vi "Generate Sine SweepV3.vi"() -> ()   [LabVIEW 2018]
uses:
  <vilib>/addons/_NISVFA/_Shared subVIs/Controls/svc_Channel Info.ctl
  <vilib>/addons/_NISVFA/_Shared subVIs/Controls/svc_Engineering Units Text Ring.ctl
  <vilib>/addons/_NISVFA/_Shared subVIs/Controls/svc_Weighting Filter Text Ring.ctl
  <vilib>/sound2/lvsound2.llb/Sound Output Task ID.ctl
  <vilib>/sound2/lvsound2.llb/Sound Input Task ID.ctl
  <vilib>/sound2/lvsound2.llb/Sound Data Format.ctl
  <vilib>/sound2/lvsound2.llb/Sampling Mode.ctl
  <vilib>/addons/Sound and Vibration/svt_Calibration/SVL Scale Voltage to EU (1 Ch).vi
  <vilib>/addons/_NISVFA/_Shared subVIs/Common/svc_Set SV Channel Info.vi
  <vilib>/addons/_NISVFA/_Shared subVIs/Common/svc_Set SV Channel Info (variant).vi
  <vilib>/addons/_NISVFA/_Shared subVIs/Common/SVL Set dB Reference (variant).vi
  <vilib>/sound2/lvsound2.llb/Sound Output Set Volume (Single).vi
  <vilib>/sound2/lvsound2.llb/Sound Output Write (DBL Single).vi
  <vilib>/sound2/lvsound2.llb/Sound Input Read (DBL).vi
  <vilib>/sound2/lvsound2.llb/Sound File Write Open.vi
  <vilib>/sound2/lvsound2.llb/Sound File Write (DBL Single).vi
  <vilib>/addons/_NISVFA/_Shared subVIs/Common/svc_Engineering Units to Unit Label.vi
  <vilib>/addons/_NISVFA/_Shared subVIs/Common/svc_Compute Scale Factor to Convert V to EU.vi
  <vilib>/addons/_NISVFA/_Shared subVIs/Common/svc_Compute Scale Factor to Convert C to EU.vi
  <vilib>/addons/_NISVFA/_Shared subVIs/Common/svc_Set dB ref if Pascal.vi
  <vilib>/addons/_NISVFA/_Shared subVIs/Common/svc_Caller VI Returned in Error Source.vi
  <vilib>/measure/maspectr.llb/FFT Power Spectrum and PSD for 1 Chan.vi
  <vilib>/addons/_NISVFA/_Baseband FFT/SVFA Frequency Response (1x1) (Mag-Phase).vi
  <vilib>/measure/macond.llb/FIR Filter for 1 Chan.vi
  <vilib>/Analysis/3filter.llb/Butterworth Filter (DBL).vi
  <vilib>/addons/_NISVFA/_Generation/SoundVib_Generation.lvlib
  <vilib>/addons/Sound and Vibration/svt_Calibration/SoundVib_Calibration.lvlib
  <vilib>/Analysis/NI_AALBase.lvlib
  <vilib>/measure/NI_MAPro.lvlib
  Program Files (x86)/National Instruments/LabVIEW 2018/examples/Sound and Vibration/SoundVib_Audio Examples.lvlib
panel:
  in  "Data Dir":path
  out "aligned signals length":i32
  out "FFT 2":cluster{"f0":dbl, "df":dbl, "magnitude":dbl[]}(graph)
  out "FFT":cluster{"f0":dbl, "df":dbl, "magnitude":dbl[]}(graph)
  in  "averaging parameters 2":T1={"averaging mode"=enum."RMS averaging", "weighting mode"=enum."Exponential", "number of averages"=10, "linear mode"=enum."Auto restart"}
  in  "FRF mode":enum16{"H1", "H2", "H3"}(ring)
  in  "view":T2={"dB On (T)"=TRUE, "unwrap phase (F)"=FALSE, "convert to degree (T)"=TRUE}
  in  "channel info Mic":T3={"sensor sensitivity"=1000.0, "engineering units"=1, "dB reference"=1.0, "custom label"="EU", "weighting filter"=0, "pregain"=0.0} {"pregain" format="%.2f"; "weighting filter" items=["Linear", "A-weighting", "B-weighting", "C-weighting", "ITU-R 468-4", "Dolby", "CCITT", "C-message", "Wb", "Wc", "Wd", "We", "Wf", "Wh", "Wj", "Wk", "Wm", "AES17 20 kHz lowpass", "AES17 40 kHz lowpass", "AES17 20 kHz highpass", "AES17 40 kHz highpass"]; "dB reference" format="%^.1e"; "engineering units" items=["custom..."=0, "V"=1, "A"=21, "C"=30, "pC"=31, "s"=32, "-"=29, "Pa"=2, "N"=20, "g"=3, "m/s^2"=4, "m/s"=5, "m"=6, "mm/s"=12, "mm"=13, "micron/s"=14, "micron"=15, "in/s^2"=7, "in/s"=8, "in"=9, "mil/s"=10, "mil"=11, "rad/s^2"=16, "rad/s"=17, "rad"=18, "deg/s^2"=26, "deg/s"=27, "deg"=28, "RPM"=22, "cycle/s^2"=23, "Hz"=24, "cycle"=25, "strain"=19]; "sensor sensitivity" format="%#_5f"}
  in  "channel info Spk":T3={"sensor sensitivity"=1000.0, "engineering units"=1, "dB reference"=1.0, "custom label"="EU", "weighting filter"=0, "pregain"=0.0} {"pregain" format="%.2f"; "weighting filter" items=["Linear", "A-weighting", "B-weighting", "C-weighting", "ITU-R 468-4", "Dolby", "CCITT", "C-message", "Wb", "Wc", "Wd", "We", "Wf", "Wh", "Wj", "Wk", "Wm", "AES17 20 kHz lowpass", "AES17 40 kHz lowpass", "AES17 20 kHz highpass", "AES17 40 kHz highpass"]; "dB reference" format="%^.1e"; "engineering units" items=["custom..."=0, "V"=1, "A"=21, "C"=30, "pC"=31, "s"=32, "-"=29, "Pa"=2, "N"=20, "g"=3, "m/s^2"=4, "m/s"=5, "m"=6, "mm/s"=12, "mm"=13, "micron/s"=14, "micron"=15, "in/s^2"=7, "in/s"=8, "in"=9, "mil/s"=10, "mil"=11, "rad/s^2"=16, "rad/s"=17, "rad"=18, "deg/s^2"=26, "deg/s"=27, "deg"=28, "RPM"=22, "cycle/s^2"=23, "Hz"=24, "cycle"=25, "strain"=19]; "sensor sensitivity" format="%#_5f"}
  out "error out 2":errorcluster
  out "FRF":cluster{"f0":dbl, "df":dbl, "magnitude":dbl[]}(graph)
  out "Waveform Mic":waveform(dbl)[](graph)
  in  "error in (no error)":errorcluster
  in  "Samples/Sec":dbl=44100.0
  in  "Amplitude":dbl(slide)=1.0 min=0.0 max=1.0 scale=0.0..1.0
  in  "device In":u32
  out "Dur(s)":dbl
  out "error out":errorcluster
  in  "device Out":u32
  in  "Duration[s]":dbl=3.0
  in  "Freq Spacing":enum16{"Linear", "Logarithmic"}(ring)=enum."Logarithmic"
  out "Waveform Out":waveform(dbl)(graph)
  in  "frequency range [Hz]":cluster{"start":dbl, "stop":dbl}={"start"=20.0, "stop"=20000.0} {"stop" format="%.2f"; "start" format="%.2f"}
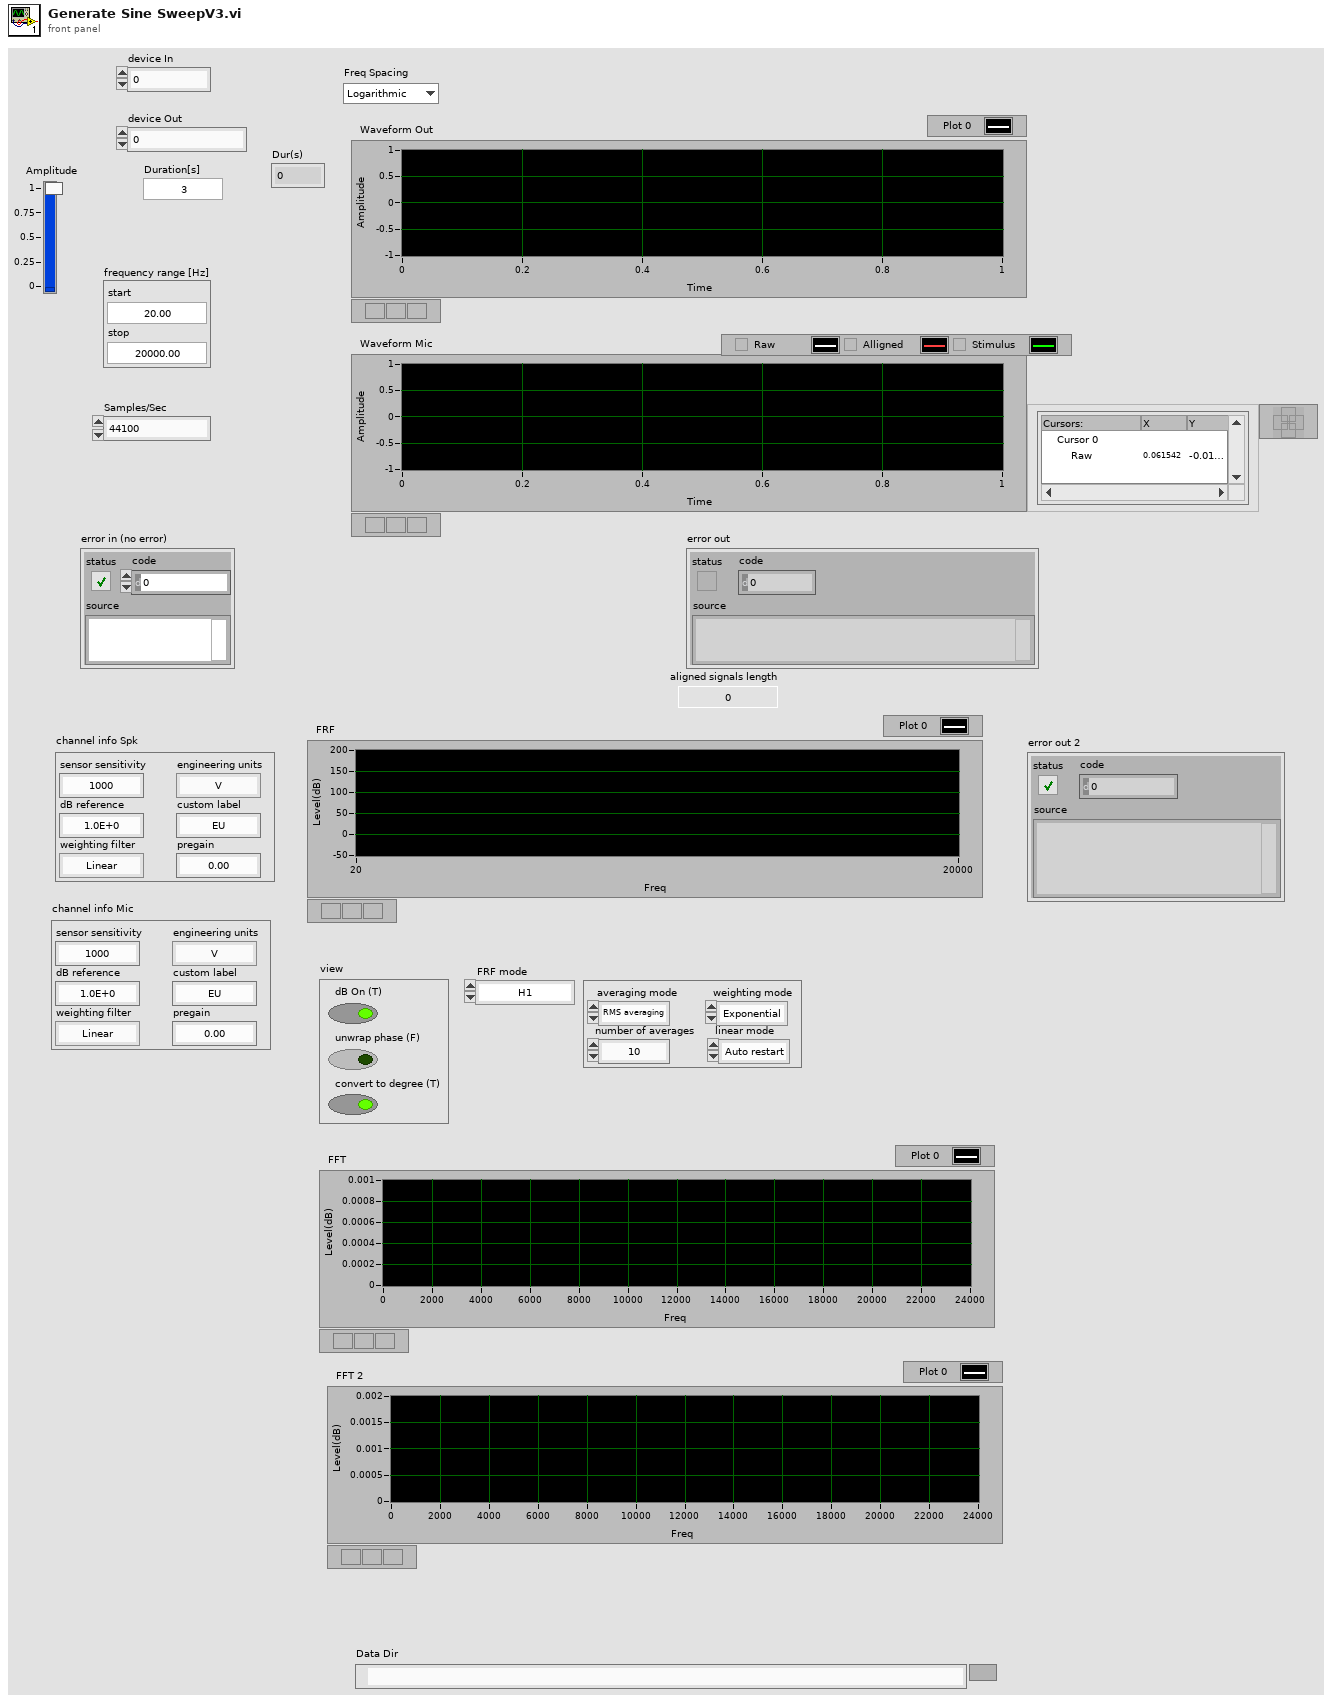
[diagram p1: front panel]
types:
  T1 = cluster{"averaging mode":enum16{"No averaging", "Vector averaging", "RMS averaging", "Peak hold"}, "weighting mode":enum16{"Linear", "Exponential"}, "number of averages":u32, "linear mode":enum16{"One shot", "Auto restart"}}
  T2 = cluster{"dB On (T)":bool, "unwrap phase (F)":bool, "convert to degree (T)":bool}
  T3 = typedef "svc_Channel Info.ctl" = cluster{"sensor sensitivity":dbl, "engineering units":T4, "dB reference":dbl, "custom label":string, "weighting filter":T5, "pregain":dbl}
  T4 = typedef "svc_Engineering Units Text Ring.ctl" = u16
  T5 = typedef "svc_Weighting Filter Text Ring.ctl" = u16
  T6 = typedef "Sound Data Format.ctl" = cluster{"sample rate (S/s)":dbl, "number of channels":i32, "bits per sample":i32}
  T7 = cluster{"Topology":enum16{"Off", "FIR by Specification", "Equi-ripple FIR", "Windowed FIR"}, "Type":enum16{"Lowpass", "Highpass", "Bandpass", "Bandstop"}, "#Taps":i32, "Lower PB":dbl, "Upper PB":dbl, "Lower SB":dbl, "Upper SB":dbl}
  T8 = typedef "Sound Input Task ID.ctl" = u32
  T9 = typedef "Sound Output Task ID.ctl" = u32
  T10 = cluster{"Start":dbl, "TaskPlay":T9, "TaskMic":T8, "SampleInfo":cluster{"Fs":dbl, "#s":u32}, "Waveform":waveform(dbl), "Samples/Sec":dbl, "Duration[s]":dbl, "Mic":waveform(dbl)[], "RcdSmpl":i32, "SoundFmt":T6}
  T11 = typedef "Sampling Mode.ctl" = i32
  T12 = typedef "Sound File Refnum.ctl" = refnum<file>
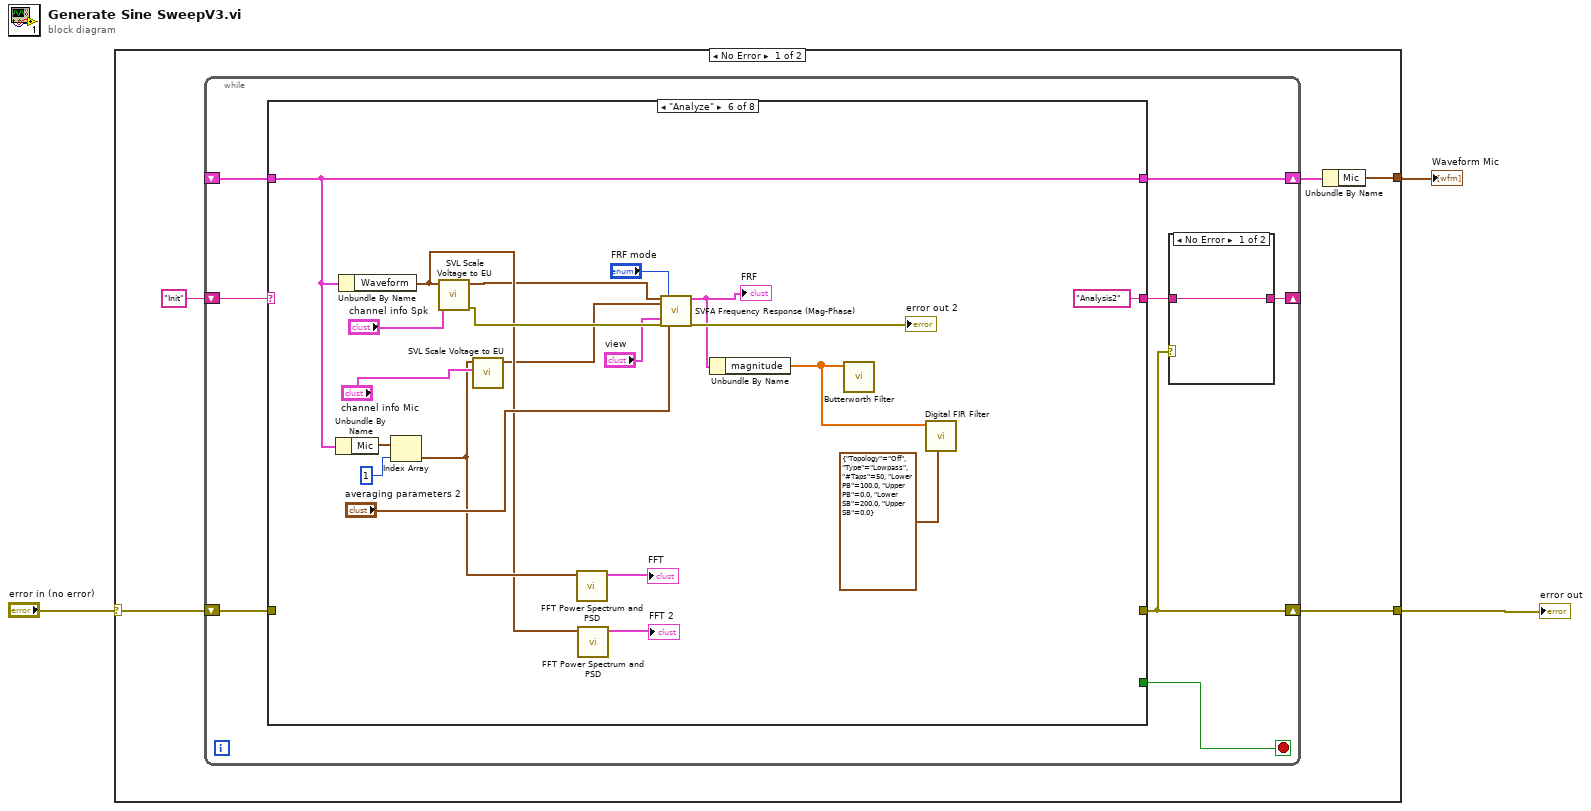
[diagram p0: block diagram]
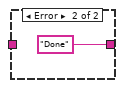
[diagram p2: hidden frame]
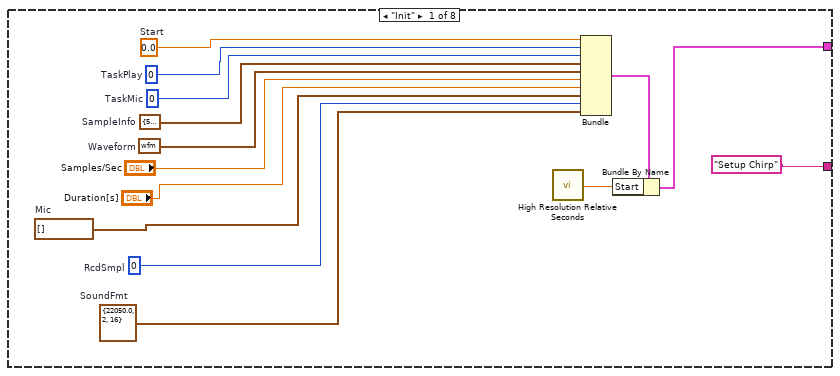
[diagram p3: hidden frame]
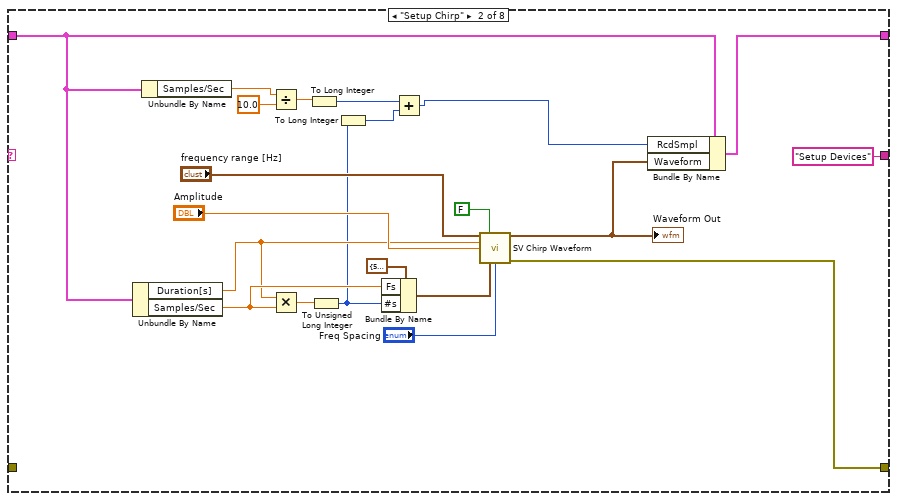
[diagram p4: hidden frame]
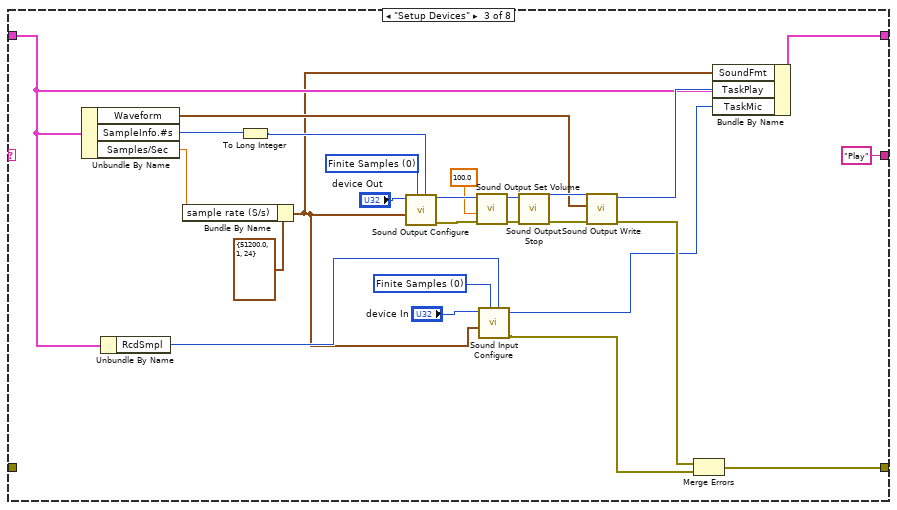
[diagram p5: hidden frame]
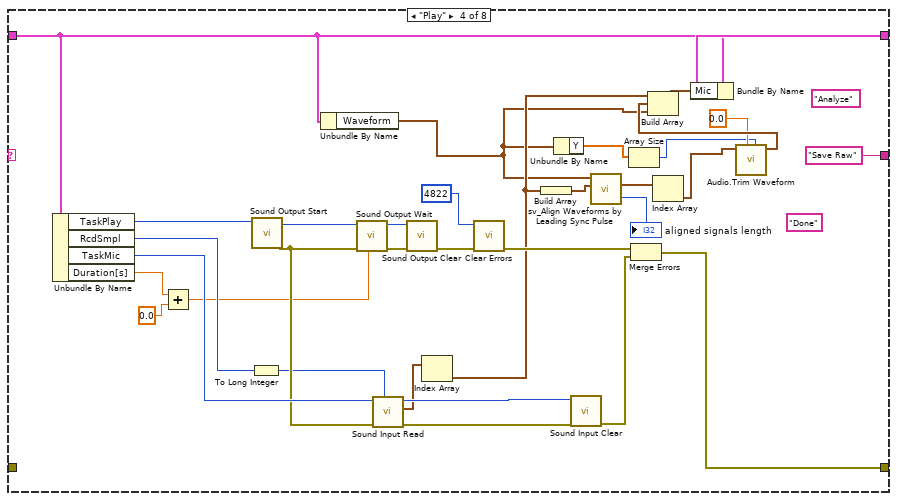
[diagram p6: hidden frame]
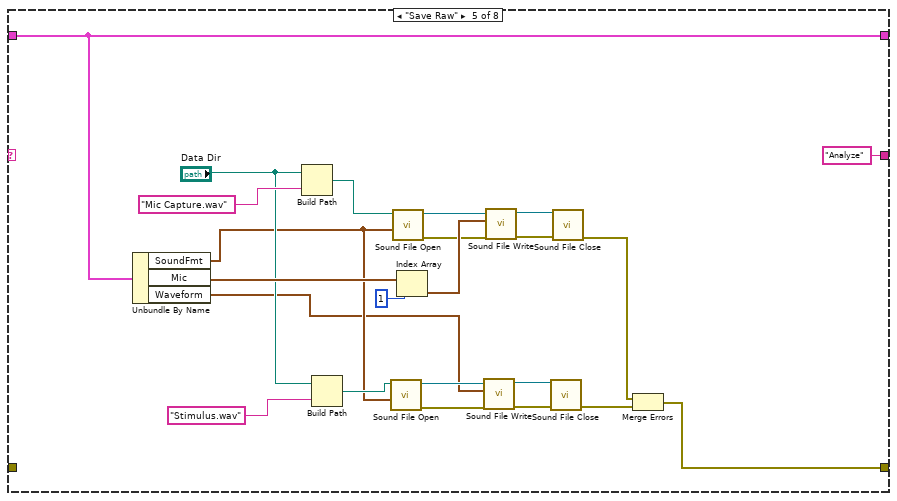
[diagram p7: hidden frame]
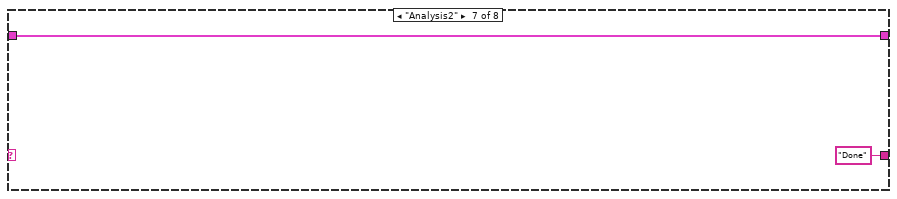
[diagram p8: hidden frame]
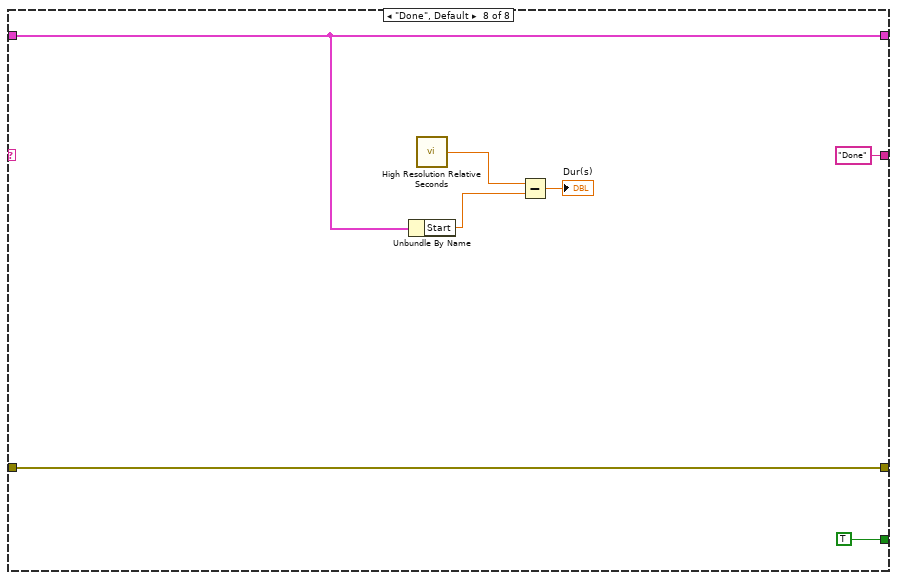
[diagram p9: hidden frame]
diagram:
  n1 = case shown="No Error" "error in (no error)" {
    selector: "error in (no error)" -> [w7 w165]
    tunnel: [w6 w165] -> w2
    tunnel: [w4 _] -> w1
    frame No Error {
      n2 = while {
        shift-right: [w12] -> _
        shift-left: "Init" -> [w16]
        shift-right: [w14] -> w5
        shift-left: _ -> [w15]
        shift-right: [w13] -> w6
        shift-left: w7 -> [w10]
        stop <- w9 stop-if-true
        n3 = case shown="\"Analyze\"" w16 {
          tunnel: w15 -> [_ w40 w56 w91 w125 w148 w156 w160]
          tunnel: ["Setup Chirp" "Setup Devices" "Play" "Save Raw" "Analyze" "Analysis2" "Done" "Done"] -> w11
          tunnel: [w24 w45 w73 w106 w125 w148 w156 w160] -> w14
          tunnel: [_ w44 w72 w107 w113 _ _ w164] -> w13
          tunnel: w10 -> [_ _ _ _ _ _ _ w164]
          tunnel: [_ _ _ _ _ _ _ TRUE] -> w9
          frame "Init" {
            w19 = T6 {"sample rate (S/s)"=22050.0, "number of channels"=2, "bits per sample"=16}  # SoundFmt
            w20 = 0  # RcdSmpl
            w21 = waveform(dbl)[] []  # Mic
            w27 = waveform(dbl) {"t0"=timestamp(0 s since 1904-01-01), "dt"=1.0, "Y"=[]}  # Waveform
            w28 = cluster{"Fs":dbl, "#s":u32} {"Fs"=51200.0, "#s"=153600}  # SampleInfo
            w29 = T8 0  # TaskMic
            w30 = T9 0  # TaskPlay
            w31 = 0.0  # Start
            n4 = call <vilib>:"High Resolution Relative Seconds.vi"() -> ("relative seconds"=w23:dbl)
            n5 = Bundle("Start"=w31, "TaskPlay"=w30, "TaskMic"=w29, "SampleInfo"=w28, "Waveform"=w27, "Samples/Sec"="Samples/Sec", "Duration[s]"="Duration[s]", "Mic"=w21, "RcdSmpl"=w20, "SoundFmt"=w19) -> (w25:T10)  [unwired: 1 in]
            n6 = Bundle By Name(cluster=w25, "Start"=w23) -> (w24:T10)
          }
          frame "Setup Chirp" {
            n7 = Unbundle By Name(w40) -> ("Duration[s]"=w41:dbl, "Samples/Sec"=w46:dbl)
            n8 = Unbundle By Name(w40) -> ("Samples/Sec"=w39:dbl)
            n9 = Divide(x=w39, y=10.0) -> (x/y=w37:dbl)
            n10 = Multiply(x=w41, y=w46) -> (x*y=w50:dbl)
            n11 = To Long Integer(number=w37) -> (32bit integer=w36:i32)
            n12 = To Unsigned Long Integer(number=w50) -> (unsigned 32bit integer=w35:u32)
            n13 = To Long Integer(number=w35) -> (32bit integer=w33:i32)
            n14 = Bundle By Name(cluster=cluster{"Fs":dbl, "#s":u32} {"Fs"=51200.0, "#s"=153600} ("sampling info"), "Fs"=w46, "#s"=w35) -> (w53:cluster{"Fs":dbl, "#s":u32})
            n15 = Add(x=w36, y=w33) -> (x+y=w34:i32)
            n16 = call <vilib>:"SV Chirp Waveform.vi"("frequency range"="frequency range [Hz]", "reset signal (F)"=FALSE, "chirp duration [s]"=w41, "amplitude"="Amplitude", "sampling info"=w53, "frequency spacing"="Freq Spacing") -> ("chirp signal"=w42:waveform(dbl), "error out"=w44:errorcluster)  [unwired: 7 in, 1 out]
            "Waveform Out" <- w42
            n17 = Bundle By Name(cluster=w40, "RcdSmpl"=w34, "Waveform"=w42) -> (w45:T10)
          }
          frame "Setup Devices" {
            w68 = T11 0 items=["Finite Samples", "Continuous Samples"] ("sample mode")
            w75 = T11 0 items=["Finite Samples", "Continuous Samples"] ("sample mode")
            n18 = Unbundle By Name(w56) -> ("Waveform"=w61:waveform(dbl), "SampleInfo.#s"=w70:u32, "Samples/Sec"=w69:dbl)
            n19 = Unbundle By Name(w56) -> ("RcdSmpl"=w55:i32)
            n20 = Bundle By Name(cluster=T6 {"sample rate (S/s)"=51200.0, "number of channels"=1, "bits per sample"=24} ("sound format"), "sample rate (S/s)"=w69) -> (w54:T6)
            n21 = To Long Integer(number=w70) -> (32bit integer=w57:i32)
            n22 = call <vilib>:"Sound Output Configure.vi"("number of samples/ch"=w57, "sample mode"=w75, "sound format"=w54, "device ID"="device Out") -> ("error out"=w79:errorcluster, "task ID"=w78:T9)  [unwired: 6 in]
            n23 = call-poly <vilib>:"Sound Output Set Volume.vi"("error in (no error)"=w79, "volume"=100.0, "task ID"=w78) -> ("error out"=w66:errorcluster, "task ID out"=w67:T9)  [unwired: 7 in]
            n24 = call <vilib>:"Sound Input Configure.vi"("number of samples/ch"=w55, "sample mode"=w68, "sound format"=w54, "device ID"="device In") -> ("error out"=w58:errorcluster, "task ID"=w59:T8)  [unwired: 6 in]
            n25 = call <vilib>:"Sound Output Stop.vi"("error in (no error)"=w66, "task ID"=w67) -> ("error out"=w64:errorcluster, "task ID out"=w65:T9)  [unwired: 8 in]
            n26 = call-poly <vilib>:"Sound Output Write.vi"("error in (no error)"=w64, "data"=w61, "task ID"=w65) -> ("error out"=w63:errorcluster, "task ID out"=w62:T9)  [unwired: 7 in]
            n27 = Merge Errors(w63, w58) -> (w72:errorcluster)
            n28 = Bundle By Name(cluster=w56, "SoundFmt"=w54, "TaskPlay"=w62, "TaskMic"=w59) -> (w73:T10)
          }
          frame "Play" {
            (unwired) "Analyze"
            (unwired) "Done"
            n29 = Unbundle By Name(w91) -> ("TaskPlay"=w105:T9, "RcdSmpl"=w100:i32, "TaskMic"=w102:T8, "Duration[s]"=w97:dbl)
            n30 = Add(x=w97, y=0.0) -> (x+y=w95:dbl)
            n31 = To Long Integer(number=w100) -> (32bit integer=w86:i32)
            n32 = call <vilib>:"Sound Output Start.vi"("task ID"=w105) -> ("error out"=w101:errorcluster, "task ID out"=w104:T9)  [unwired: 9 in]
            n33 = Unbundle By Name(w91) -> ("Waveform"=w82:waveform(dbl))
            n34 = call <vilib>:"Sound Output Wait.vi"("timeout (sec)"=w95, "error in (no error)"=w101, "task ID"=w104) -> ("error out"=w112:errorcluster, "task ID out"=w108:T9)  [unwired: 7 in]
            n35 = call-poly <vilib>:"Sound Input Read.vi"("number of samples/ch"=w86, "error in (no error)"=w101, "task ID"=w102) -> ("error out"=w111:errorcluster, "data"=w98:waveform(dbl)[], "task ID out"=w110:T8)  [unwired: 6 in]
            n36 = call <vilib>:"Sound Output Clear.vi"("error in (no error)"=w112, "task ID"=w108) -> ("error out"=w94:errorcluster)  [unwired: 9 in]
            n37 = Index Array(array=w98) -> (element=w88:waveform(dbl))  [unwired: 1 in]
            n38 = call <vilib>:"Clear Errors.vi"("error in (no error)"=w94, "specific error code to clear (0: all)"=4822) -> ("error out"=w93:errorcluster)  [unwired: 4 in, 1 out]
            n39 = Build Array(w88) -> (w90:waveform(dbl)[])
            n40 = Unbundle By Name(w82) -> ("Y"=w81:dbl[])
            n41 = call <vilib>:"Sound Input Clear.vi"("error in (no error)"=w111, "task ID"=w110) -> ("error out"=w109:errorcluster)  [unwired: 9 in]
            n42 = call "sv_Align Waveforms by Leading Sync Pulse.vi"("response signals"=w90, "alignment reference signal"=w82) -> ("aligned signals"=w89:waveform(dbl)[], "aligned signals length"=→"aligned signals length":i32)  [unwired: 5 in, 3 out]
            n43 = Array Size(array=w81) -> (size(s)=w80:i32)
            n44 = Merge Errors(w93, w109) -> (w107:errorcluster)
            n45 = Index Array(array=w89) -> (element=w85:waveform(dbl))  [unwired: 1 in]
            n46 = call "Audio.Trim Waveform.vi"("Len"=w80, "Max Delay"=0.0, "Data In"=w85) -> ("Data Out"=w84:waveform(dbl))  [unwired: 8 in]
            n47 = Build Array(w88, w84, w82) -> (w103:waveform(dbl)[])
            n48 = Bundle By Name(cluster=w91, "Mic"=w103) -> (w106:T10)
          }
          frame "Save Raw" {
            n49 = Unbundle By Name(w125) -> ("SoundFmt"=w117:T6, "Mic"=w135:waveform(dbl)[], "Waveform"=w116:waveform(dbl))
            n50 = Build Path(base path="Data Dir", name or relative path="Mic Capture.wav") -> (appended path=w132:path)
            n51 = Build Path(base path="Data Dir", name or relative path="Stimulus.wav") -> (appended path=w118:path)
            n52 = call-poly <vilib>:"Sound File Open.vi"("sound format"=w117, "path"=w118) -> ("error out"=w123:errorcluster, "sound file refnum"=w121:T12)  [unwired: 8 in]
            n53 = call-poly <vilib>:"Sound File Open.vi"("sound format"=w117, "path"=w132) -> ("error out"=w128:errorcluster, "sound file refnum"=w131:T12)  [unwired: 8 in]
            n54 = Index Array(array=w135, index=1) -> (element=w129:waveform(dbl))
            n55 = call-poly <vilib>:"Sound File Write.vi"("error in (no error)"=w123, "data"=w116, "sound file refnum"=w121) -> ("error out"=w124:errorcluster, "sound file refnum out"=w122:T12)  [unwired: 7 in]
            n56 = call-poly <vilib>:"Sound File Write.vi"("error in (no error)"=w128, "data"=w129, "sound file refnum"=w131) -> ("error out"=w127:errorcluster, "sound file refnum out"=w130:T12)  [unwired: 7 in]
            n57 = call <vilib>:"Sound File Close.vi"("error in (no error)"=w124, "sound file refnum"=w122) -> ("error out"=w115:errorcluster)  [unwired: 9 in]
            n58 = call <vilib>:"Sound File Close.vi"("error in (no error)"=w127, "sound file refnum"=w130) -> ("error out"=w114:errorcluster)  [unwired: 9 in]
            n59 = Merge Errors(w114, w115) -> (w113:errorcluster)
          }
          frame "Analyze" {
            n60 = Unbundle By Name(w148) -> ("Mic"=w154:waveform(dbl)[])
            n61 = Unbundle By Name(w148) -> ("Waveform"=w141:waveform(dbl))
            n62 = Index Array(array=w154, index=1) -> (element=w144:waveform(dbl))
            n63 = call-poly <vilib>:"SVL Scale Voltage to EU.vi"("channel info"="channel info Spk", "signal [V]"=w141) -> ("error out"=w152:errorcluster, "scaled signal [EU]"=w140:waveform(dbl))  [unwired: 7 in, 1 out]
            n64 = call-poly <vilib>:"SVL Scale Voltage to EU.vi"("channel info"="channel info Mic", "signal [V]"=w144) -> ("scaled signal [EU]"=w139:waveform(dbl))  [unwired: 7 in, 2 out]
            n65 = call-poly <vilib>:"FFT Power Spectrum and PSD.vi"("time signal"=w144) -> ("Power Spectrum / PSD"=→"FFT":cluster{"f0":dbl, "df":dbl, "magnitude":dbl[]})  [unwired: 7 in, 3 out]
            n66 = call-poly <vilib>:"FFT Power Spectrum and PSD.vi"("time signal"=w141) -> ("Power Spectrum / PSD"=→"FFT 2":cluster{"f0":dbl, "df":dbl, "magnitude":dbl[]})  [unwired: 7 in, 3 out]
            n67 = call-poly <vilib>:"SVFA Frequency Response (Mag-Phase).vi"("stimulus signal X [EUx]"=w140, "response signal Y [EUy]"=w139, "view"="view", "error in (no error)"=w152, "FRF mode"="FRF mode", "averaging parameters"="averaging parameters 2") -> ("magnitude [dB EUy/EUx]"=w138:cluster{"f0":dbl, "df":dbl, "magnitude":dbl[]}, "error out"=→"error out 2":errorcluster)  [unwired: 5 in, 7 out]
            "FRF" <- w138
            n68 = Unbundle By Name(w138) -> ("magnitude"=w137:dbl[])
            n69 = call-poly <vilib>:"Butterworth Filter.vi"("X"=w137) -> ()  [unwired: 7 in, 2 out]
            n70 = call-poly <vilib>:"Digital FIR Filter.vi"("FIR filter specifications"=T7 {"Topology"=enum."Off", "Type"=enum."Lowpass", "#Taps"=50, "Lower PB"=100.0, "Upper PB"=0.0, "Lower SB"=200.0, "Upper SB"=0.0}, "signal in"=w137) -> ()  [unwired: 7 in, 3 out]
          }
          frame "Analysis2" {
          }
          frame "Done", Default {
            n71 = Unbundle By Name(w160) -> ("Start"=w159:dbl)
            n72 = call <vilib>:"High Resolution Relative Seconds.vi"() -> ("relative seconds"=w161:dbl)
            n73 = Subtract(x=w161, y=w159) -> (x-y=→"Dur(s)":dbl)
          }
        }
        n74 = case shown="No Error" w13 {
          tunnel: [w17 "Done"] -> w12
          tunnel: w11 -> [w17 _]
          frame No Error {
          }
          frame Error {
          }
        }
      }
      n75 = Unbundle By Name(w5) -> ("Mic"=w4:waveform(dbl)[])
    }
    frame Error {
    }
  }
  "error out" <- w2
  "Waveform Mic" <- w1
